vi "Picker Upper.vi"(0 "State Control":enum16{"Open", "Run", "End"}(ring)=enum."Run", 1 "Encoder":dbl, 5 "Up":bool, 7 "Down":bool, 9 "Top limit":bool, 11 "Bottom Limit":bool, 12 "Down break":dbl=2000.0 format="%#_13g") -> (4 "Fully up?":bool, 15 "Fully down?":bool)   [LabVIEW 2013]
uses:
  <vilib>/Rock Robotics/SystemInterfaces/DIO/FPGA_DIOPWMChannel.ctl
  <vilib>/Rock Robotics/WPI/MotorControl/WPI_MotorControlOpen Talon.vi
panel:
  in  "Up break":dbl=5.0
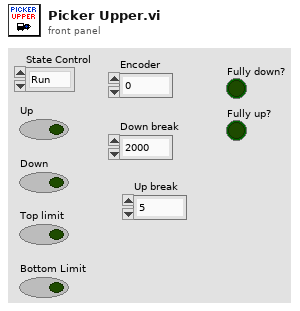
[diagram p1: front panel]
types:
  T1 = typedef "FPGA_DIOPWMChannel.ctl" = enum8{"PWM 1", "PWM 2", "PWM 3", "PWM 4", "PWM 5", "PWM 6", "PWM 7", "PWM 8", "PWM 9", "PWM 10", "Invalid"}
  T2 = typedef "WPI_MotorControlDeviceRef.ctl" = cluster{"DeviceStatus":errorcluster, "Type":enum16{"PWM", "CAN"}, "PWM":cluster{"Digital Module":T3, "PWM Channel":T1, "DeadBand":T4}, "CAN":cluster{"Device Number":u8, "Control Mode":T5, "Semaphore":T6, "Max Vout":dbl}, "Invert":bool, "TransformRef":T7, "InvTransformRef":T7}
  T3 = typedef "FPGA_TypedefDigitalModule.ctl" = enum16{"Digital Module 1", "Digital Module 2"}
  T4 = typedef "WPI_PWMDeadband.ctl" = cluster{"Name":string, "maxPositivePwm":i32, "minPositivePwm":i32, "centerPwm":i32, "maxNegativePwm":i32, "minNegativePwm":i32, "angularRange":u16}
  T5 = typedef "WPI_CANJaguar_ControlMode.ctl" = enum8{"Percent VBus", "Current", "Speed", "Position", "Voltage"}
  T6 = typedef "Semaphore RefNum" = refnum<k1>
  T7 = typedef "WPI_PWMTransform_ConPane.ctl" = refnum<vi>
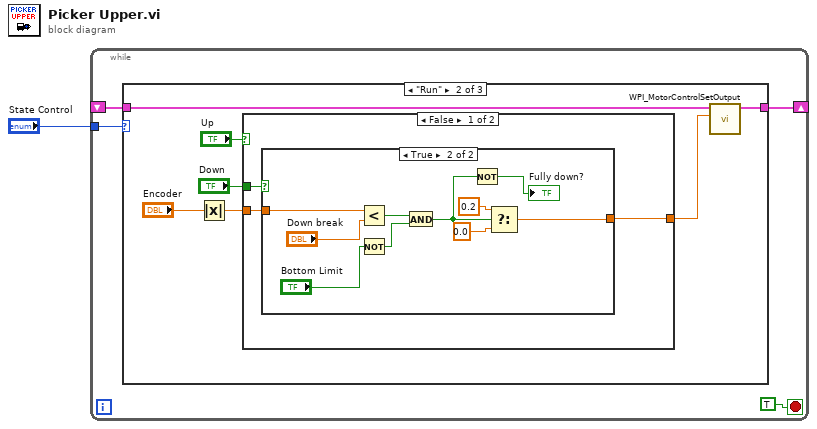
[diagram p0: block diagram]
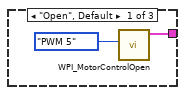
[diagram p2: hidden frame]
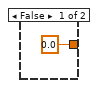
[diagram p3: hidden frame]
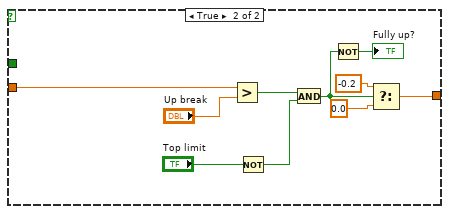
[diagram p4: hidden frame]
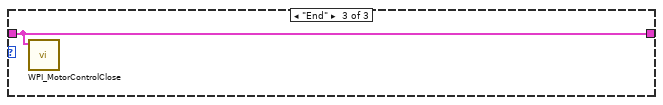
[diagram p5: hidden frame]
diagram:
  n1 = while {
    shift-right: [w2] -> _
    shift-left: _ -> [w5]
    tunnel: "State Control" -> [w4]
    stop <- TRUE stop-if-true
    n2 = case shown="\"Run\"" w4 {
      tunnel: w5 -> [_ w14 w39]
      tunnel: [w6 w13 w39] -> w2
      frame "Open", Default {
        n3 = call-poly <vilib>:"WPI_MotorControlOpen.vi"("PWM Channel"=FPGA_DIOPWMChannel."PWM 5") -> ("MotorControlDeviceRef"=w6:T2)  [unwired: 9 in, 1 out]
      }
      frame "Run" {
        n4 = Absolute Value(x="Encoder") -> (abs(x)=w10:dbl)
        n5 = case shown="False" "Up" {
          tunnel: "Down" -> [w17 _]
          tunnel: w10 -> [w16 w33]
          tunnel: [w15 w35] -> w12
          frame False {
            n6 = case shown="True" w17 {
              tunnel: w16 -> [_ w27]
              tunnel: [0.0 ("f") w23] -> w15
              frame False {
              }
              frame True {
                n7 = Less?(x=w27, y="Down break") -> (x < y?=w22:bool)
                n8 = Not(x="Bottom Limit") -> (.not. x?=w28:bool)
                n9 = And(x=w22, y=w28) -> (x .and. y?=w20:bool)
                n10 = Not(x=w20) -> (.not. x?=→"Fully down?":bool)
                n11 = Select(t=0.2 ("Numeric"), s=w20, f=0.0) -> (s? t:f=w23:dbl)
              }
            }
          }
          frame True {
            n12 = Greater?(x=w33, y="Up break") -> (0:w34:bool)
            n13 = Not(x="Top limit") -> (.not. x?=w38:bool)
            n14 = And(x=w34, y=w38) -> (x .and. y?=w30:bool)
            n15 = Not(x=w30) -> (.not. x?=→"Fully up?":bool)
            n16 = Select(t=-0.2, s=w30, f=0.0) -> (s? t:f=w35:dbl)
          }
        }
        n17 = call <vilib>:"WPI_MotorControlSetOutput.vi"("Output"=w12, "MotorControlDevRef"=w14) -> ("MotorControlDevRef"=w13:T2)  [unwired: 7 in, 2 out]
      }
      frame "End" {
        n18 = call <vilib>:"WPI_MotorControlClose.vi"("MotorControlDevRef"=w39) -> ()  [unwired: 10 in, 1 out]
      }
    }
  }
